vi "oax_gsPolar Plot.vi"() -> ()   [LabVIEW 2017]
doc: "This is Order Analysis Toolkit demo VI."
uses:
  <vilib>/addons/Sound and Vibration/Order Analysis/Tach Process/SoundVib_TachProcess.lvlib
  <vilib>/addons/Sound and Vibration/Order Analysis/Resample Order Tracking/SoundVib_OrderTracking.lvlib
  <vilib>/Waveform/WDTOps.llb/WDT Waveform Duration DBL.vi
  <vilib>/addons/Sound and Vibration/Order Analysis/Data Presentation/SoundVib_OAVisualization.lvlib
  <vilib>/addons/Sound and Vibration/Order Analysis/Data Presentation/SVX Polar Plot (1 Channel).vi
  <vilib>/addons/Sound and Vibration/Order Analysis/Data Presentation/SubVIs/OAT MCM Channel Property.ctl
  <vilib>/addons/_XControls/Polar Plot/SVX Polar Plot.xctl
panel:
  out "Polar Plot":T1(xcontrol)
  in  "bandwidth [order]":dbl format="%.2f"
  in  "buffer settings":cluster{"buffer mode":u16, "buffer size":dbl}={"buffer mode"=0, "buffer size"=100.0} {"buffer mode" items=["Infinite length", "Last block data", "Custom"]}
  in  "X axis selection":u16(ring)=2 items=["Time", "Revolution", "RPM"]
  in  "order to display":dbl=1.0 format="%.2f"
  in  "channel settings":T2 {"probe angle [deg]" max=360 step=1; "shaft rotating direction" items=["CCW", "CW"]}
  in  "Select Data":i32(listbox)
  in  "STOP":bool
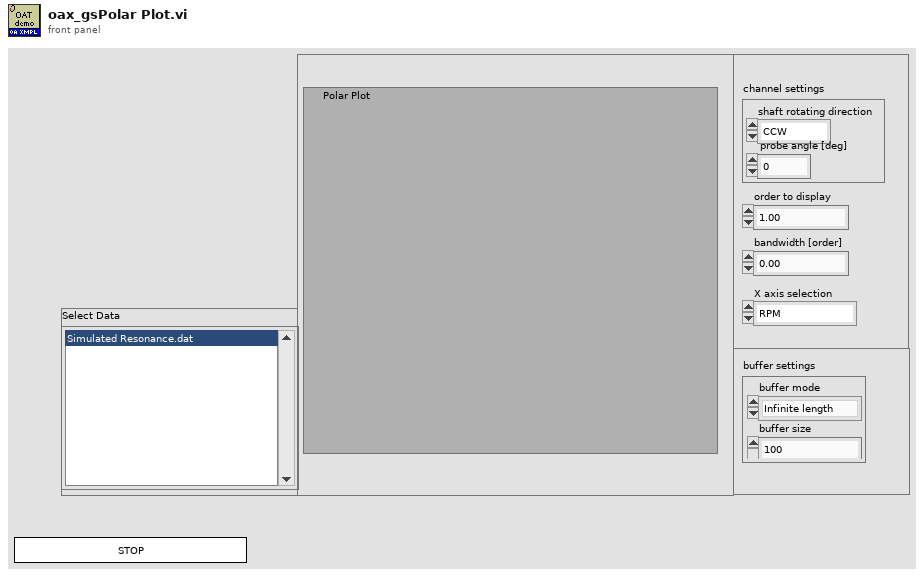
[diagram p1: front panel]
types:
  T1 = cluster{"magnitude":dbl[], "phase":dbl[], "time/rev/RPM":dbl[], "attribute":variant}[][]
  T2 = cluster{"shaft rotating direction":u16, "probe angle [deg]":u16}
  T3 = typedef "OAT MCM Channel Property.ctl" = cluster{"direction":u16, "probe angle [deg]":u16, "pair":u16}
  T4 = cluster{"dB on? (T)":bool, "unwrap phase? (T)":bool, "unit in degree? (T)":bool}
  T5 = typedef "SoundVib_TachProcess.lvlib/speed profile.ctl" = cluster{"time [s]":dbl[], "speed [RPM]":dbl[]}
  T6 = typedef "svc_Resampled Channel Info.ctl" = cluster{"channel name":string, "description":string, " channel info":T7}
  T7 = typedef "svc_Channel Info.ctl" = cluster{"sensor sensitivity":dbl, "engineering units":T8, "dB reference":dbl, "custom label":string, "weighting filter":T9, "pregain":dbl}
  T8 = typedef "svc_Engineering Units Text Ring.ctl" = u16
  T9 = typedef "svc_Weighting Filter Text Ring.ctl" = u16
  T10 = typedef "OAT Position Info.ctl" = cluster{"positions [s]":dbl[], "samples/rev":dbl}
  T11 = cluster{"time/rev/rpm":dbl[], "magnitude":dbl[]}[]
  T12 = typedef "svc_Spectrum Info.ctl" = cluster{"channel name":string, "description":string, "x-axis units":T13, "spectral info":cluster{"spectrum type":T14, "linear/dB":enum16{"linear", "dB"}, "window":u16, "window size":i32, "FFT size":i32}, "engineering units":T8, "custom label":string, "dB reference [EU]":dbl, "peak units":enum16{"rms", "peak", "peak-peak"}, "weighting filter":T9, "spectral density?":bool, "unit label":string, "spectrum skewed?":bool, "complimentary spectrum units":T15}
  T13 = typedef "svc_X-Axis Units.ctl" = u16
  T14 = typedef "svc_Spectrum Type.ctl" = enum16{"FFT Spectrum [complex]", "Amplitude [Magnitude]", "Power [Magnitude^2]", "Cross Spectrum [complex]", "Frequency Response [Complex]"}
  T15 = typedef "svc_Complimentary Spectrum Units.ctl" = enum16{"none", "radians", "degrees", "cycles", "imaginary"}
  T16 = cluster{"pulse / rev":i32, "threshold (auto)":dbl, "slope (Rising)":u16}
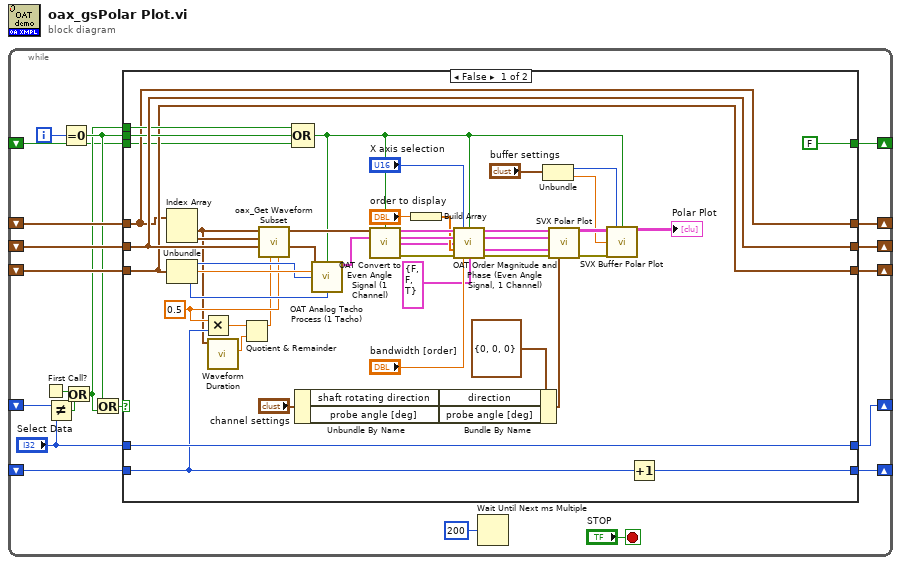
[diagram p0: block diagram]
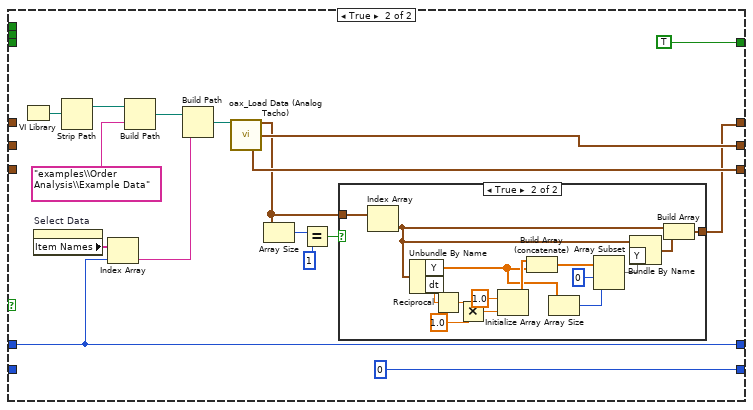
[diagram p2: hidden frame]
diagram:
  n1 = while {
    shift-right: [w17] -> _
    shift-left: _ -> [w18]
    shift-right: [w15] -> _
    shift-left: _ -> [w21]
    shift-right: [w14] -> _
    shift-left: _ -> [w19]
    shift-right: [w13] -> _
    shift-left: _ -> [w12]
    shift-right: [w3] -> _
    shift-left: _ -> [w4]
    shift-right: [w2] -> _
    shift-left: _ -> [w1]
    i -> [w11]
    stop <- "STOP" stop-if-true
    n2 = First Call?() -> (First Call?: T/F=w7:bool)
    n3 = Not Equal?(x=w18, y="Select Data") -> (x != y?=w6:bool)
    n4 = Equal To 0?(x=w11) -> (x = 0?=w10:bool)
    n5 = Or(x=w7, y=w6) -> (x .or. y?=w5:bool)
    n6 = Or(x=w10, y=w5) -> (x .or. y?=w9:bool)
    n7 = case shown="False" w9 {
      tunnel: w21 -> [w49 _]
      tunnel: w19 -> [w66 _]
      tunnel: [w67 w84] -> w17
      tunnel: "Select Data" -> [w67 w84]
      tunnel: [w49 w69] -> w15
      tunnel: [w66 w82] -> w14
      tunnel: [w60 w81] -> w13
      tunnel: w12 -> [w60 _]
      tunnel: w5 -> [w64 _]
      tunnel: w10 -> [w63 _]
      tunnel: w4 -> [w54 _]
      tunnel: [w56 0] -> w3
      tunnel: [FALSE TRUE] -> w2
      tunnel: w1 -> [w48 _]
      frame False {
        w55 = 0.5 ("y")
        n8 = Index Array(array=w49) -> (element #1=w53:waveform(dbl), element #2=w61:waveform(dbl))  [unwired: 2 in]
        n9 = Unbundle(w60) -> ("pulse / rev"=w58:i32, "threshold (auto)"=w59:dbl, "slope (Rising)"=w57:u16)
        n10 = Multiply(x=w55, y=w54) -> (x*y=w51:dbl)
        n11 = call-poly <vilib>:"Waveform Duration.vi"("waveform in"=w53) -> ("duration"=w52:dbl)  [unwired: 8 in, 2 out]
        n12 = Quotient & Remainder(x=w51, y=w52) -> (x-y*floor(x/y)=w50:dbl)  [unwired: 1 out]
        n13 = call <vilib>:"oax_Get Waveform Subset.vi"("duration"=w55, "start index"=w50, "Tach Signal"=w66, "Vibration Signal Y"=w61, "Vibration Signal X"=w53) -> ("Tach Signal out"=w65:waveform(dbl), "Vibration Signal X out"=w62:waveform(dbl))  [unwired: 3 in, 2 out]
        n14 = Compound Arithmetic op=OR(w64, w63, w48) -> (w26:bool)
        n15 = Unbundle By Name("channel settings") -> ("shaft rotating direction"=w31:u16, "probe angle [deg]"=w30:u16)
        n16 = call <vilib>:"OAT Analog Tacho Process (1 Tacho).vi"("analog tacho signal"=w65, "reset? (F)"=w26, "threshold (auto)"=w59, "pulse/revolution (1)"=w58, "slope (Rising)"=w57) -> ("speed profile"=w68:T5)  [unwired: 6 in, 4 out]
        n17 = call <vilib>:"OAT Convert to Even Angle Signal (1 Channel).vi"("scaled signal [EU]"=w62, "reset? (F)"=w26, "speed profile"=w68) -> ("even-angle signal"=w46:cluster{"r0":dbl, "dr":dbl, "Y":dbl[]}, "even-angle channel info"=w45:T6, "even-angle position info"=w40:T10, "error out"=w44:errorcluster)  [unwired: 8 in, 1 out]
        n18 = Build Array("order to display") -> (w42:dbl[])
        n19 = Bundle By Name(cluster=T3 {"direction"=0, "probe angle [deg]"=0, "pair"=0} ("channel properties"), "direction"=w31, "probe angle [deg]"=w30) -> (w29:T3)
        n20 = call <vilib>:"OAT Order Magnitude and Phase (Even Angle Signal, 1 Channel).vi"("even-angle signal"=w46, "x-axis selection"="X axis selection", "reset? (F)"=w26, "even-angle channel info"=w45, "even-angle position info"=w40, "orders to compute (1.0)"=w42, "error in (no error)"=w44, "bandwidth [order]"="bandwidth [order]", "view"=T4 {"dB on? (T)"=FALSE, "unwrap phase? (T)"=FALSE, "unit in degree? (T)"=TRUE}) -> ("magnitudes [RMS]"=w37:T11, "phases [phase lag]"=w36:cluster{"time/rev/rpm":dbl[], "phase":dbl[]}[], "magnitude info"=w35:T12, "error out"=w34:errorcluster)  [unwired: 1 in, 2 out]
        n21 = Unbundle("buffer settings") -> ("buffer mode"=w24:u16, "buffer size"=w23:dbl)
        n22 = call-poly <vilib>:"SVX Polar Plot.vi"("magnitudes [RMS]"=w37, "phases [phase lag]"=w36, "magnitude info"=w35, "error in (no error)"=w34, "channel properties"=w29) -> ("polar plot"=w28:T1, "error out"=w27:errorcluster)  [unwired: 8 in, 1 out]
        n23 = call <vilib>:"SVX Buffer Polar Plot.vi"("polar plot data in"=w28, "buffer mode"=w24, "reset? (F)"=w26, "buffer size"=w23, "error in (no error)"=w27) -> ("polar plot data out"=→"Polar Plot":T1)  [unwired: 9 in, 1 out]
        n24 = Increment(x=w54) -> (x+1=w56:i32)
      }
      frame True {
        n25 = VI Library() -> (path=w77:path)
        n26 = property on="Select Data" class="LstBox (strict)"() -> ("Item Names"=w85:string[])  [unwired: 2 in, 2 out]
        n27 = Strip Path(path=w77) -> (stripped path=w76:path)  [unwired: 1 out]
        n28 = Index Array(array=w85, index=w84) -> (element=w79:string)
        n29 = Build Path(base path=w76, name or relative path="examples\\Order Analysis\\Example Data") -> (appended path=w80:path)
        n30 = Build Path(base path=w80, name or relative path=w79) -> (appended path=w78:path)
        n31 = call <vilib>:"oax_Load Data (Analog Tacho).vi"("Data Path In"=w78) -> ("vibration data"=w70:waveform(dbl)[], "analog tacho signal"=w82:waveform(dbl), "tacho info"=w81:T16)  [unwired: 8 in, 4 out]
        n32 = Array Size(array=w70) -> (size(s)=w73:i32)
        n33 = Equal?(x=w73, y=1) -> (x = y?=w71:bool)
        n34 = case shown="True" w71 {
          tunnel: w70 -> [w86 w101]
          tunnel: [w86 w100] -> w69
          frame False {
          }
          frame True {
            n35 = Index Array(array=w101) -> (element=w99:waveform(dbl))  [unwired: 1 in]
            n36 = Unbundle By Name(w99) -> ("Y"=w88:dbl[], "dt"=w97:dbl)
            n37 = Reciprocal(x=w97) -> (1/x=w96:dbl)
            n38 = Multiply(x=w96, y=1.0) -> (x*y=w94:dbl)
            n39 = Initialize Array(1.0 ("element"), w94) -> (w90:dbl[])
            n40 = Build Array (concatenate)(w90, w88) -> (w92:dbl[])
            n41 = Array Size(array=w88) -> (size(s)=w89:i32)
            n42 = Array Subset(array=w92, index=0, length=w89) -> (w87:dbl[])
            n43 = Bundle By Name(cluster=w99, "Y"=w87) -> (w98:waveform(dbl))
            n44 = Build Array(w99, w98) -> (w100:waveform(dbl)[])
          }
        }
      }
    }
    n45 = Wait Until Next ms Multiple(millisecond multiple=u32 200) -> ()  [unwired: 1 out]
  }
